vi "vision_pc.vi"() -> ()   [LabVIEW 2017]
uses:
  <vilib>/userdefined/High Color/IMAQdx.ctl
  <vilib>/vision/driver/NI_Vision_Acquisition_Software.lvlib
panel:
  out "зеленый":bool
  in  "stop":bool
  out "Image":T1(plugin-control)
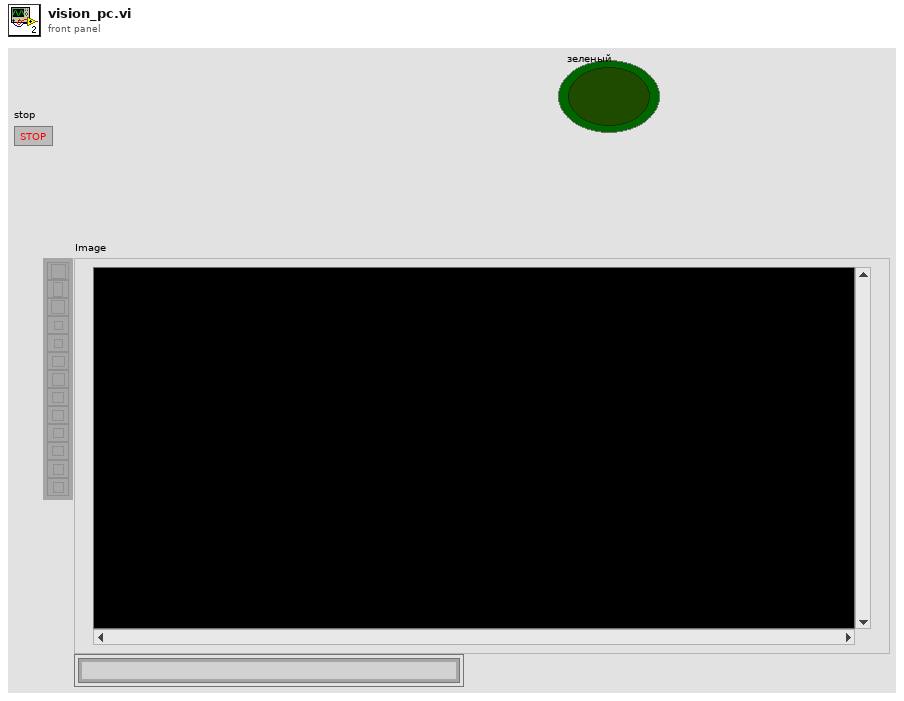
[diagram p1: front panel]
types:
  T1 = typedef "IMAQ Image.ctl" = refnum<image>
  T2 = typedef "IMAQdx.ctl" = refnum<k21>
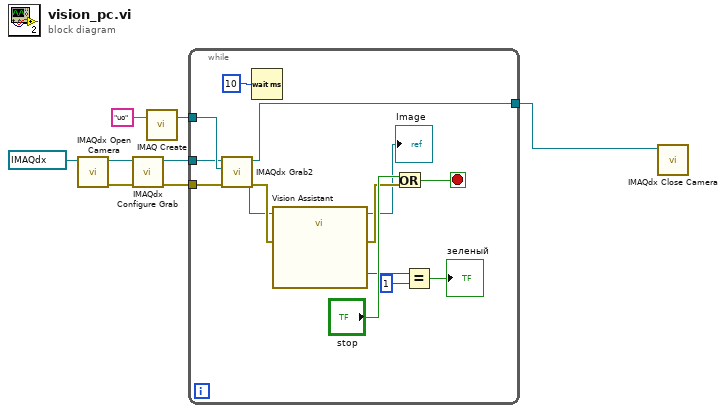
[diagram p0: block diagram]
diagram:
  n1 = call <vilib>:"IMAQdx Open Camera.vi"("Session In"=T2 "cam0") -> ("error out"=w8:errorcluster, "Session Out"=w5:T2)  [unwired: 9 in]
  n2 = call <vilib>:"IMAQdx Configure Grab.vi"("error in"=w8, "Session In"=w5) -> ("error out"=w7:errorcluster, "Session Out"=w4:T2)  [unwired: 8 in]
  n3 = call "IMAQ Create"("Image Name"="uo") -> ("New Image"=w6:T1)  [unwired: 4 in, 1 out]
  n4 = while {
    tunnel: w7 -> [w22]
    tunnel: w6 -> [w20]
    tunnel: w4 -> [w19]
    tunnel: [w18] -> w3
    stop <- w21 stop-if-true
    n5 = call <vilib>:"IMAQdx Grab2.vi"("error in"=w22, "Image In"=w20, "Session In"=w19) -> ("error out"=w14:errorcluster, "Image Out"=w12:T1, "Session Out"=w18:T2)  [unwired: 5 in, 1 out]
    n6 = Wait (ms)(milliseconds to wait=u32 10) -> ()  [unwired: 1 out]
    n7 = call "Vision Assistant"("Image In"=w12, "error in"=w14) -> ("Image Out"=→"Image":T1, "Number of Matches (Color Pattern Matching 1)"=w11:i32, "error out"=w15:errorcluster)  [unwired: 23 in]
    n8 = Or(x="stop", y=w15) -> (x .or. y?=w21:bool)
    n9 = Equal?(x=w11, y=1) -> (x = y?=→"зеленый":bool)
  }
  n10 = call <vilib>:"IMAQdx Close Camera.vi"("Session In"=w3) -> ()  [unwired: 10 in, 1 out]
